vi "SCI_Tx_Pack.vi"(9 "数据有效":bool, 10 "数据类型":u16 format="%x", 11 "数据":u16 format="%x") -> (1 "CRC余数":u16 format="%x", 3 "数据包输出":T1 {"包头" format="%02x"; "数据低8位" format="%02x"; "数据低高8位" format="%02x"; "数据类型" items=["VOID"]; "CRC余数" format="%02x"})   [LabVIEW 2015]
uses:
  SCI_DataPck.ctl
  SCI_DataType.ctl
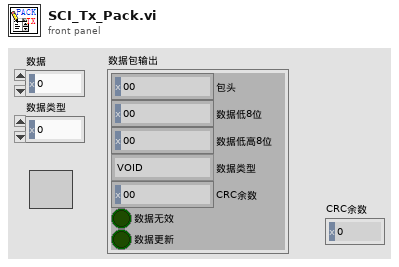
[diagram p1: front panel]
types:
  T1 = typedef "SCI_DataPck.ctl" = cluster{"包头":u16, "数据低8位":u16, "数据低高8位":u16, "数据类型":T2, "CRC余数":u16, "数据无效":bool, "数据更新":bool}
  T2 = typedef "SCI_DataType.ctl" = u16
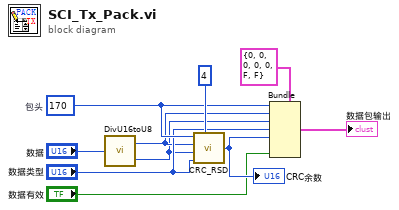
[diagram p0: block diagram]
diagram:
  w9 = u16 170  # 包头
  n1 = call "DivU16toU8.vi"("Uint16_in"="数据") -> ("Uint8L_out"=w6:u8, "Uint8H_out"=w5:u8)
  n2 = call "CRC_RSD.vi"("BYTE 0"=w9, "BYTE 1"=w6, "BYTE 2"=w5, "BYTE 3"="数据类型", "Number of BYTE"=4) -> ("RSD"=w4:u16)
  "CRC余数" <- w4
  n3 = Bundle(cluster=T1 {"包头"=0, "数据低8位"=0, "数据低高8位"=0, "数据类型"=0, "CRC余数"=0, "数据无效"=FALSE, "数据更新"=FALSE}, "包头"=w9, "数据低8位"=w6, "数据低高8位"=w5, "数据类型"="数据类型", "CRC余数"=w4, "数据更新"="数据有效") -> (→"数据包输出":T1)  [unwired: 1 in]
